vi "pack tcp packet.vi"(7 "tcp-message-type":T1=enum."cmd", 11 "String":string) -> (3 "TCP Pack":string)   [LabVIEW 2020, in "CSM-TCP-Router.lvlib"]
uses:
  CSM-TCP-Router.lvlib
  typedef/tcp-msg type.ctl
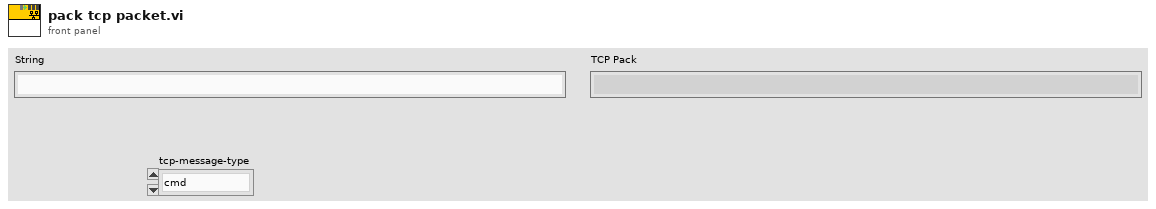
[diagram p1: front panel]
types:
  T1 = typedef "CSM-TCP-Router.lvlib/tcp-msg type.ctl" = enum8{"info", "error", "cmd", "resp", "async-resp", "status", "interrupt"}
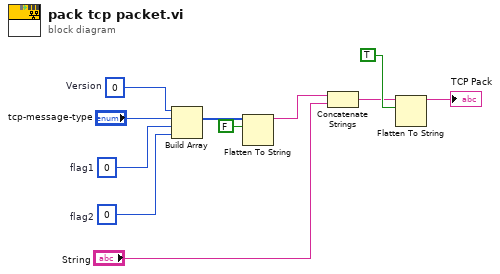
[diagram p0: block diagram]
diagram:
  w1 = u8 0  # Version
  w2 = u8 0  # flag2
  w3 = u8 0  # flag1
  n1 = Build Array(w1, "tcp-message-type", w3, w2) -> (w4:u8[])
  n2 = Flatten To String(anything=w4, prepend array or string size? (T)=FALSE) -> (data string=w5:string)  [unwired: 1 in, 3 out]
  n3 = Concatenate Strings(w5, "String") -> (w8:string)
  n4 = Flatten To String(anything=w8, prepend array or string size? (T)=TRUE) -> (data string=→"TCP Pack":string)  [unwired: 1 in, 3 out]
